vi "Flatten Dependencies To String Array.vi"(3 "User Deps":T1[](array[typedef])) -> (1 "User Deps":string[][](array[string]))   [LabVIEW 2011, in "LMH-Toolbox.lvlib" / "LMH-Installer Tools.lvlib"]
uses:
  LMH-Installer Tools.lvlib
  Type Defs/User Dependency.ctl
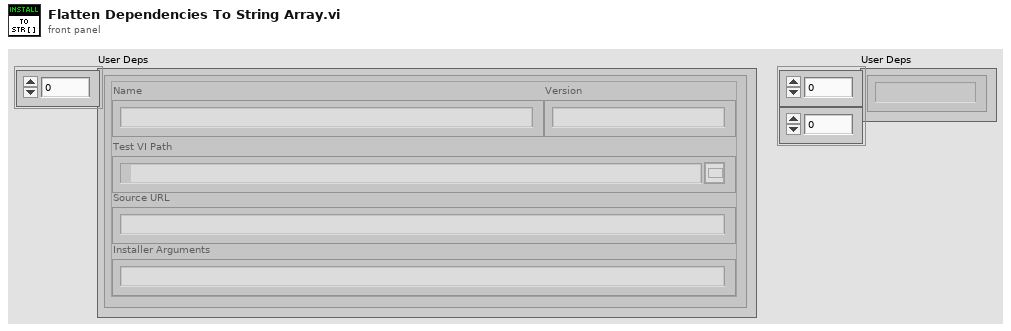
[diagram p1: front panel]
types:
  T1 = typedef "LMH-Toolbox.lvlib/LMH-Installer Tools.lvlib/User Dependency.ctl" = cluster{"Name":string, "Version":string, "Test VI Path":path, "Source URL":string, "Installer Arguments":string}
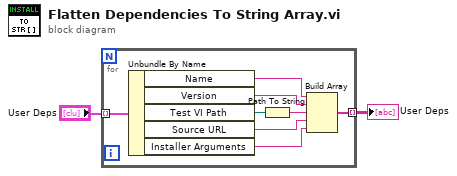
[diagram p0: block diagram]
diagram:
  n1 = for {
    tunnel: "User Deps" -> [w10] mode=indexing
    tunnel: [w4] -> w1 mode=indexing
    n2 = Unbundle By Name(w10) -> ("Name"=w8:string, "Version"=w6:string, "Test VI Path"=w9:path, "Source URL"=w5:string, "Installer Arguments"=w3:string)
    n3 = Path To String(path=w9) -> (string=w7:string)
    n4 = Build Array(w8, w6, w7, w5, w3) -> (w4:string[])
  }
  "User Deps" <- w1
